vi "Add Buffer Channels.vi"(1 "byte order":T3, 4 "channels":T4[](array[typedef]) {"core"."string offset" format="%d bytes"}, 6 "Decimation":u64, 8 "error in (no error)":errorcluster, 9 "buffer descriptor":T1={"buffer type"=enum."Engine", "plugin id"=-1, "group id"=-1, "transfer id"=-1, "offset"=0, "length"=-1}, 10 "parent tag":string, 11 "Application Data In":T8={"Item Tree Control"=refnum, "Top-Level VI"=refnum, "menu reference"=refnum, "queue"=refnum, "Stop Pointer"=refnum, "Buffer Variant"=variant, "server ID"=refnum, "framework tag"="", "Values"=refnum, "Hex"=refnum, "ASCII"=refnum, "lines visible"=0, "values padding"=0, "current buffer data"={"decimation"=0, "avg bandwidth"=0.0, "channels"=[], "byte order"=enum."little-endian", "buffer descriptor"={"buffer type"=enum."Engine", "plugin id"=0, "group id"=0, "transfer id"=0, "offset"=0, "length"=0}, "values channels"={"index"=0, "count"=0, "engine offset"=0}, "select start offset"=18446744073709551615, "select end offset"=0, "channel index"=-1}, "Framework Configuration"=refnum} {"current buffer data"."channels"."configuration"."string offset" format="%d bytes"; "current buffer data"."avg bandwidth" format="%.0g bytes"}) -> (0 "error out":errorcluster, 3 "Application Data out":T8={"Item Tree Control"=refnum, "Top-Level VI"=refnum, "menu reference"=refnum, "queue"=refnum, "Stop Pointer"=refnum, "Buffer Variant"=variant, "server ID"=refnum, "framework tag"="", "Values"=refnum, "Hex"=refnum, "ASCII"=refnum, "lines visible"=0, "values padding"=0, "current buffer data"={"decimation"=0, "avg bandwidth"=0.0, "channels"=[], "byte order"=enum."little-endian", "buffer descriptor"={"buffer type"=enum."Engine", "plugin id"=0, "group id"=0, "transfer id"=0, "offset"=0, "length"=0}, "values channels"={"index"=0, "count"=0, "engine offset"=0}, "select start offset"=18446744073709551615, "select end offset"=0, "channel index"=-1}, "Framework Configuration"=refnum} {"current buffer data"."channels"."configuration"."string offset" format="%d bytes"; "current buffer data"."avg bandwidth" format="%.0g bytes"})   [LabVIEW 2017, in "DSF Core.lvlib"]
uses:
  DSF Core.lvlib
  Main VI/Application Data.ctl
  <vilib>/NI/Memory Manager/Classes/Pointer/Pointer.lvclass
  Classes/Configuration/Core/Framework/Framework Configuration.lvclass
  Buffer Reader/Queue Data.ctl
  Buffer Reader/Buffer Data.ctl
  Classes/Configuration/Core/Transfer/Channel Configuration.ctl
  Typedefs/Core Channel Configuration.ctl
  Typedefs/DSF Data Type.ctl
  Typedefs/DSF Settings Info.ctl
  Typedefs/DSF Byte Order.ctl
  Classes/Thread/Data Server/DSF Buffer Subset Descriptor.ctl
  Typedefs/DSF Buffer Type.ctl
  Main VI/Values Channels.ctl
  Typedefs/DSF Engine Channel Configuration.ctl
  ID to Tree Items/Tree Item Type.ctl
  Classes/Framework/Framework.lvclass
  Classes/Configuration/Core/Channel/Channel Configuration.lvclass
  Classes/Configuration/Core/Transfer/Transfer Configuration.lvclass
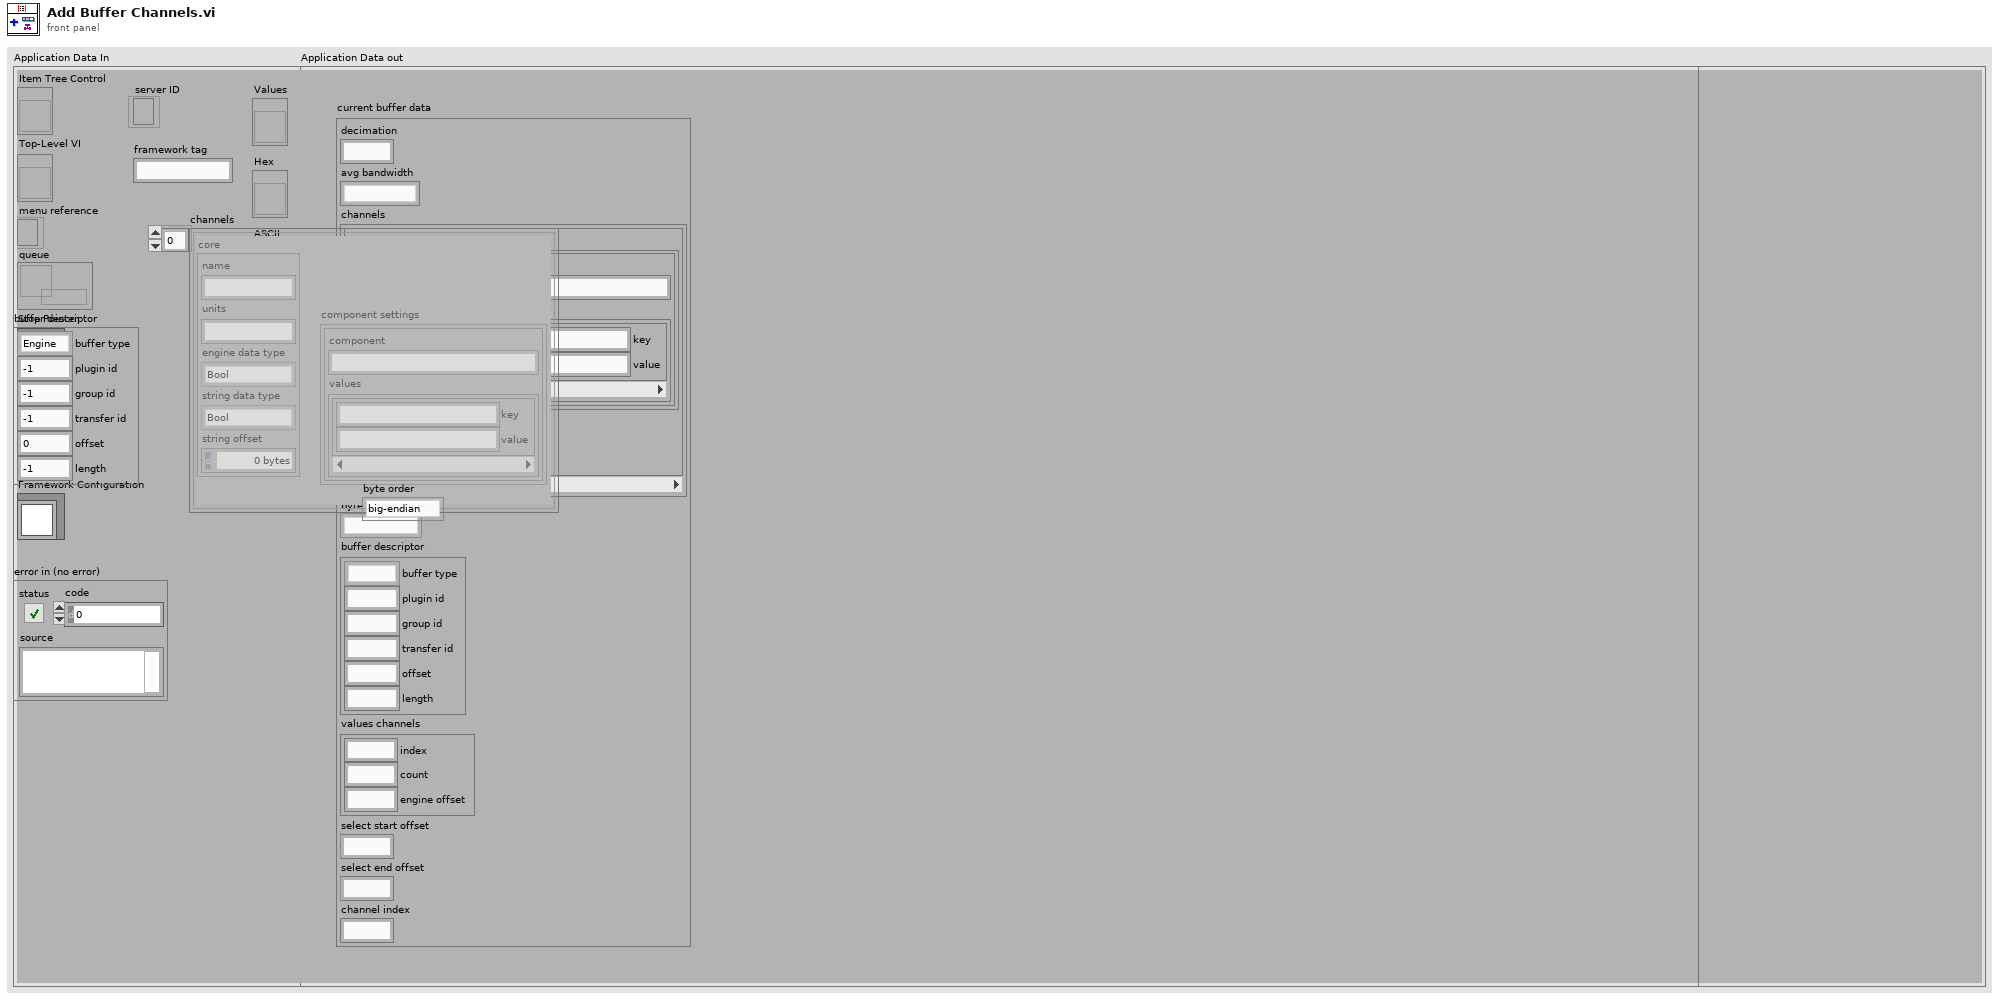
[diagram p1: front panel]
types:
  T1 = typedef "DSF Core.lvlib/DSF Buffer Subset Descriptor.ctl" = cluster{"buffer type":T2, "plugin id":i32, "group id":i32, "transfer id":i32, "offset":u64, "length":i64}
  T2 = typedef "DSF Core.lvlib/DSF Buffer Type.ctl" = enum16{"Engine", "String"}
  T3 = typedef "DSF Core.lvlib/DSF Byte Order.ctl" = enum8{"big-endian", "little-endian"}
  T4 = typedef "DSF Core.lvlib/DSF Engine Channel Configuration.ctl" = cluster{"core":T5, "component settings":T7[]}
  T5 = typedef "DSF Core.lvlib/Channel Configuration.lvclass/Core Channel Configuration.ctl" = cluster{"name":string, "units":string, "engine data type":T6, "string data type":T6, "string offset":u64}
  T6 = typedef "DSF Core.lvlib/DSF Data Type.ctl" = enum8{"Bool", "SGL", "DBL", "I8", "I16", "I32", "I64", "U8", "U16", "U32", "U64"}
  T7 = typedef "DSF Core.lvlib/DSF Settings Info.ctl" = cluster{"component":string, "values":cluster{"key":string, "value":string}[]}
  T8 = typedef "DSF Core.lvlib/Application Data.ctl" = cluster{"Item Tree Control":refnum<vi>, "Top-Level VI":refnum<vi>, "menu reference":refnum<k9>, "queue":refnum<queue>, "Stop Pointer":refnum<class "Pointer.lvclass">, "Buffer Variant":variant, "server ID":refnum<k5>, "framework tag":string, "Values":refnum<vi>, "Hex":refnum<vi>, "ASCII":refnum<vi>, "lines visible":i32, "values padding":i32, "current buffer data":T9, "Framework Configuration":refnum<class "Framework Configuration.lvclass">}
  T9 = typedef "DSF Core.lvlib/Buffer Data.ctl" = cluster{"decimation":u64, "avg bandwidth":dbl, "channels":T10[], "byte order":T3, "buffer descriptor":T1, "values channels":T11, "select start offset":u64, "select end offset":u64, "channel index":i32}
  T10 = typedef "DSF Core.lvlib/Transfer Configuration.lvclass/Channel Configuration.ctl" = cluster{"configuration":T5, "component settings":T7[]}
  T11 = typedef "DSF Core.lvlib/Values Channels.ctl" = cluster{"index":i32, "count":i32, "engine offset":u64}
  T12 = typedef "DSF Core.lvlib/Tree Item Type.ctl" = enum16{"Framework", "Plugin Group", "Plugin", "Group", "Transfer", "Buffer", "Channel"}
  T13 = typedef "DSF Core.lvlib/Tree Item.ctl" = cluster{"Left Cell String":string, "Child Text":string[], "Child Tag":string, "Glyph Index":i32}
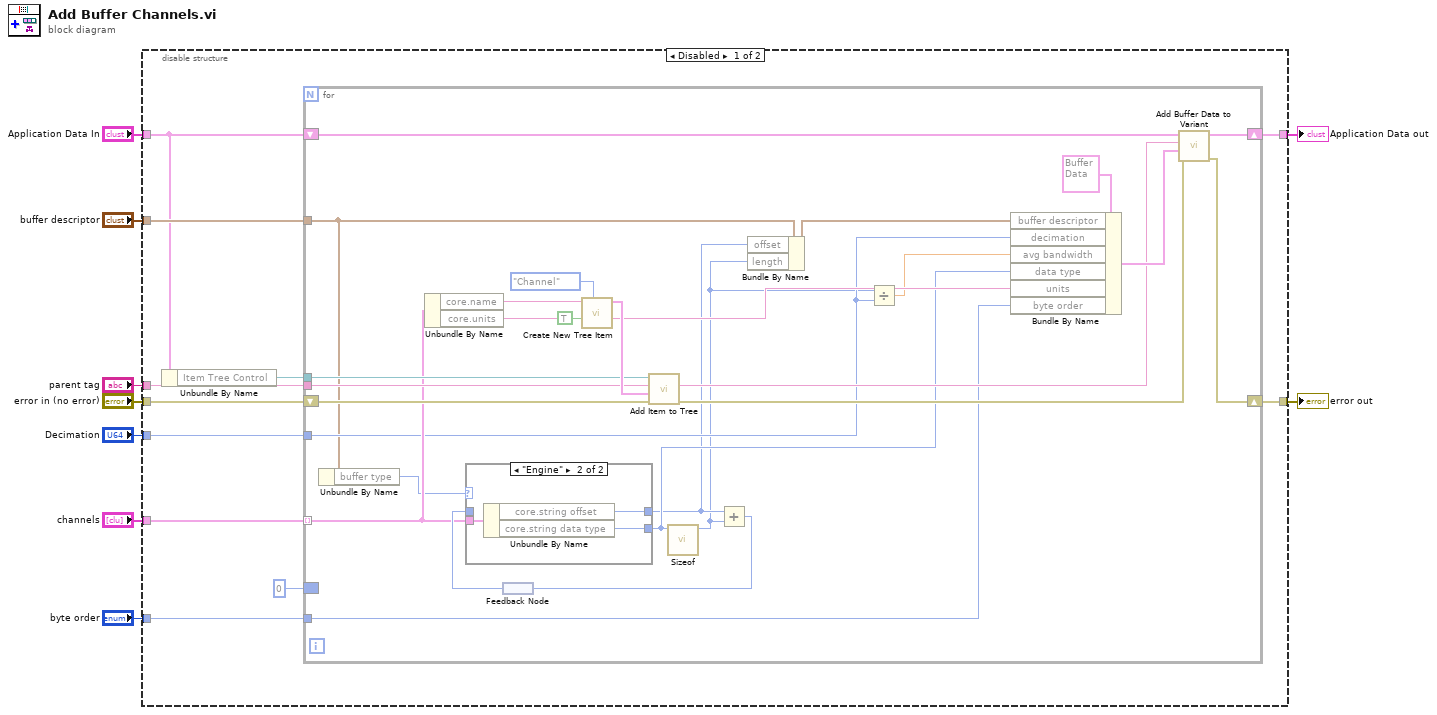
[diagram p0: block diagram]
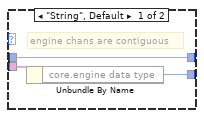
[diagram p2: hidden frame]
diagram:
  n1 = disable-structure shown="Disabled" {
    disable-tunnel: [w20 _] -> w9
    disable-tunnel: [w19 _] -> w8
    disable-tunnel: "error in (no error)" -> [w18 _]
    disable-tunnel: "parent tag" -> [w16 _]
    disable-tunnel: "Decimation" -> [w15 _]
    disable-tunnel: "channels" -> [w14 _]
    disable-tunnel: "byte order" -> [w12 _]
    disable-tunnel: "buffer descriptor" -> [w11 _]
    disable-tunnel: "Application Data In" -> [w10 _]
    frame Disabled {
      n2 = Unbundle By Name(w10) -> ("Item Tree Control"=w17:refnum<vi>)
      n3 = for {
        tunnel: w17 -> [w38]
        tunnel: w16 -> [w37]
        tunnel: w15 -> [w28]
        shift-right: [w45] -> w19
        shift-left: w18 -> [w42]
        shift-right: [w46] -> w20
        shift-left: w10 -> [w23]
        tunnel: w14 -> [w33] mode=indexing
        border: u64 0 -> [_]
        tunnel: w12 -> [w29]
        tunnel: w11 -> [w22]
        n4 = Unbundle By Name(w22) -> ("buffer type"=w21:T2)
        n5 = Unbundle By Name(w33) -> ("core.name"=w32:string, "core.units"=w31:string)
        n6 = feedback #1() -> (w36:u64)
        n7 = case shown="\"Engine\"" w21 {
          tunnel: w33 -> [w50 w53]
          tunnel: [w49 w52] -> w30
          tunnel: [w48 w51] -> w26
          tunnel: w36 -> [w48 _]
          frame "String", Default {
            # "engine chans are contiguous"
            n8 = Unbundle By Name(w50) -> ("core.engine data type"=w49:T6)
          }
          frame "Engine" {
            n9 = Unbundle By Name(w53) -> ("core.string offset"=w51:u64, "core.string data type"=w52:T6)
          }
        }
        n10 = call "Create New Tree Item.vi"("Item Type"=Tree_Item_Type."Channel", "found?"=TRUE, "Left Cell String"=w32) -> ("Item"=w39:T13)  [unwired: 7 in, 1 out]
        n11 = call "Add Item to Tree.vi"("error in (no error)"=w42, "Item"=w39, "parent tag"=w37, "TreeControl in"=w38) -> ("error out"=w47:errorcluster, "new item tag"=w34:string)  [unwired: 5 in, 1 out]
        n12 = call "Sizeof.vi"("data type"=w30) -> ("size in bytes"=w25:u64)  [unwired: 9 in, 1 out]
        n13 = Add(x=w26, y=w25) -> (x+y=w35:u64)
        n14 = feedback-in #1(w35) -> ()
        n15 = Bundle By Name(cluster=w22, "offset"=w26, "length"=w25) -> (w27:T1)
        n16 = Divide(x=w25, y=w28) -> (x/y=w24:dbl)
        n17 = Bundle By Name(cluster=T9 {"decimation"=0, "avg bandwidth"=0.0, "channels"=[], "byte order"=enum."big-endian", "buffer descriptor"={"buffer type"=enum."Engine", "plugin id"=0, "group id"=0, "transfer id"=0, "offset"=0, "length"=0}, "values channels"={"index"=0, "count"=0, "engine offset"=0}, "select start offset"=18446744073709551615, "select end offset"=0, "channel index"=-1} ("Buffer data"), "buffer descriptor"=w27, "decimation"=w28, "avg bandwidth"=w24, "data type"=w30, "units"=w31, "byte order"=w29) -> (w44:T9)
        n18 = call "Add Buffer Data to Variant.vi"("error in (no error)"=w47, "Buffer data"=w44, "tag"=w34, "Application Data In in"=w23) -> ("error out"=w45:errorcluster, "Application Data In out"=w46:T8)  [unwired: 6 in]
      }
    }
    frame Enabled {
    }
  }
  "error out" <- w8
  "Application Data out" <- w9
